vi "Halo Loop.vi"   [LabVIEW 2013]
uses:
  Robot Global Data.vi
  <vilib>/Rock Robotics/WPI/Solenoid/Deprecated/WPI_SolenoidSetBool.vi
types:
  T1 = typedef "WPI_SolenoidDevRef.ctl" = cluster{"DevStatus":errorcluster, "Solenoid Module":T2, "Forward Solenoid Channel":T3, "Reverse Solenoid Channel":T3}
  T2 = typedef "FPGA_TypedefSolenoidModule.ctl" = enum16{"Solenoid Module 1", "Solenoid Module 2"}
  T3 = typedef "WPI_SolenoidChannel.ctl" = enum8{"Solenoid 1", "Solenoid 2", "Solenoid 3", "Solenoid 4", "Solenoid 5", "Solenoid 6", "Solenoid 7", "Solenoid 8", "Invalid"}
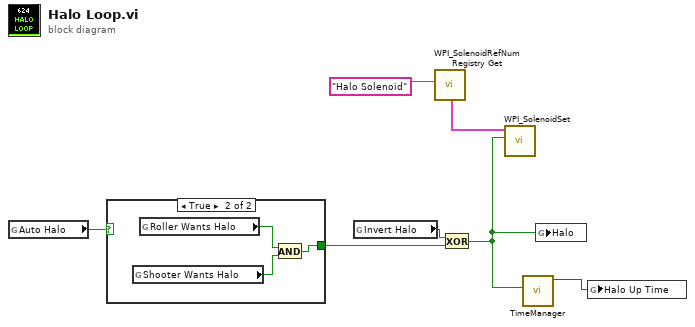
[diagram p0: block diagram]
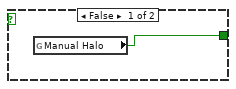
[diagram p2: hidden frame]
diagram:
  n1 = global read "Robot Global Data.vi" "Auto Halo"() -> (w5:bool)
  n2 = case shown="True" w5 {
    tunnel: [w8 w9] -> w3
    frame False {
      n3 = global read "Robot Global Data.vi" "Manual Halo"() -> (w8:bool)
    }
    frame True {
      n4 = global read "Robot Global Data.vi" "Shooter Wants Halo"() -> (w10:bool)
      n5 = global read "Robot Global Data.vi" "Roller Wants Halo"() -> (w11:bool)
      n6 = And(x=w11, y=w10) -> (x .and. y?=w9:bool)
    }
  }
  n7 = global read "Robot Global Data.vi" "Invert Halo"() -> (w1:bool)
  n8 = call <vilib>:"WPI_SolenoidRefNum Registry Get.vi"("refnum name"="Halo Solenoid") -> ("SolenoidDevRef"=w6:T1)  [unwired: 9 in, 1 out]
  n9 = Exclusive Or(1:w3, 2:w1) -> (0:w2:bool)
  n10 = call-poly <vilib>:"WPI_SolenoidSet.vi"("Value"=w2, "SolenoidDevRef"=w6) -> ()  [unwired: 8 in, 2 out]
  n11 = call "TimeManager.vi"("Reset?"=w2) -> ("Time Since Reset"=w4:u32)  [unwired: 9 in, 1 out]
  n12 = global write "Robot Global Data.vi" "Halo"(w2) -> ()
  n13 = global write "Robot Global Data.vi" "Halo Up Time"(w4) -> ()
